vi "NI VeriStand - Reconnect to System.vi"(6 "Deploy System Definition (T)":bool=TRUE, 7 "Calibration File":path, 8 "error in (no error)":errorcluster, 9 "Timeout (60000 ms)":u32=60000, 10 "Target":string, 11 "WorkspaceManager in":T1) -> (0 "error out":errorcluster, 3 "WorkspaceManager out":T1)   [LabVIEW 2020, in "NI_VS Workspace ExecutionAPI.lvlib"]
doc: "Reconnects the VeriStand Gateway to a particular target."
uses:
  <vilib>/NI VeriStand/Execution/Workspace/NI_VS Workspace ExecutionAPI.lvlib
  <vilib>/NI VeriStand/Execution/Workspace/WorkspaceAPI.ctl
  NationalInstruments.VeriStand.ClientAPI
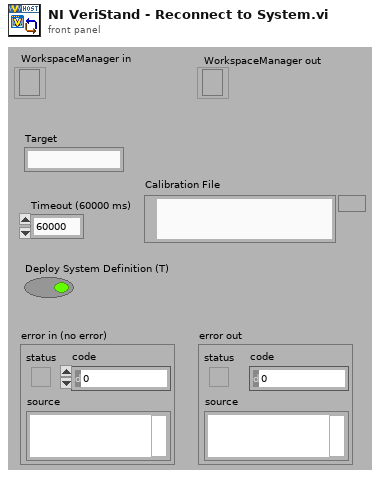
[diagram p1: front panel]
types:
  T1 = typedef "NI_VS Workspace ExecutionAPI.lvlib/WorkspaceAPI.ctl" = refnum<k24>
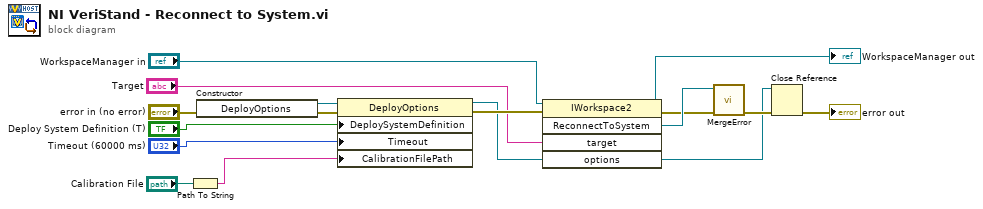
[diagram p0: block diagram]
diagram:
  n1 = Path To String(path="Calibration File") -> (string=w1:string)
  n2 = constructor class="DeployOptions"(error in="error in (no error)") -> (reference out=w12:refnum<k24>, error out=w8:errorcluster)  [unwired: 2 in, 1 out]
  n3 = property class="DeployOptions"(reference=w12, error in=w8, "DeploySystemDefinition"="Deploy System Definition (T)", "Timeout"="Timeout (60000 ms)", "CalibrationFilePath"=w1) -> (reference out=w4:refnum<k24>, error out=w7:errorcluster)
  n4 = invoke class="IWorkspace2" method="ReconnectToSystem"(reference="WorkspaceManager in", error in=w7, "target"="Target", "options"=w4) -> (reference out=→"WorkspaceManager out":T1, error out=w13:errorcluster, "ReconnectToSystem"=w14:refnum<k24>)  [unwired: 1 in, 2 out]
  n5 = call <vilib>:"MergeError.vi"("error in (no error)"=w13, "Error"=w14) -> ("error out"=w6:errorcluster)  [unwired: 9 out]
  n6 = Close Reference(reference=w4, error in (no error)=w6) -> (error out=→"error out":errorcluster)
